vi "Read Tag.vi"(8 "error in (no error)":errorcluster, 11 "TreeEditCellMsg in":refnum<class "TreeEditCellMsg.lvclass">) -> (0 "error out":errorcluster, 2 "Tag":string, 3 "TreeEditCellMsg out":refnum<class "TreeEditCellMsg.lvclass">)   [LabVIEW 2015, in "ActorEvents.lvlib" / "TreeEditCellMsg.lvclass"]
uses:
  TreeEditCellMsg.lvclass
  TreeEditCellMsg.lvclass/TreeEditCellMsg.ctl
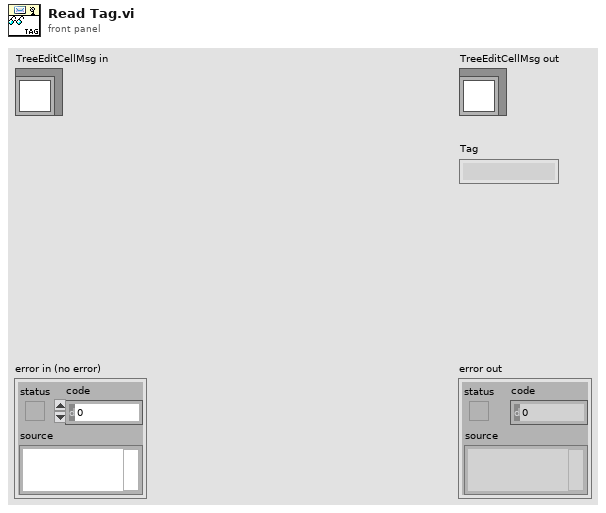
[diagram p1: front panel]
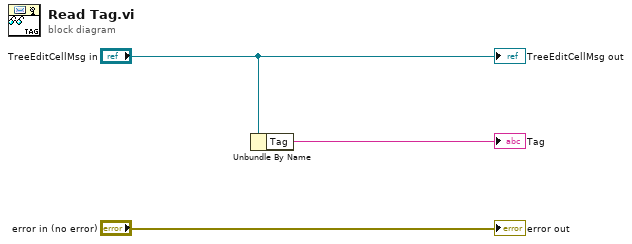
[diagram p0: block diagram]
diagram:
  n1 = Unbundle By Name("TreeEditCellMsg in") -> ("Tag"=→"Tag":string)
  "error out" <- "error in (no error)"
  "TreeEditCellMsg out" <- "TreeEditCellMsg in"
